vi "myXi_ReshapeArray.vi"(9 "width":i32, 10 "height":i32, 11 "acquisition frame":T1) -> (3 "output array":u16[][](array[numeric]))   [LabVIEW 2018]
uses:
  typedef/AcquisitionFrame.ctl
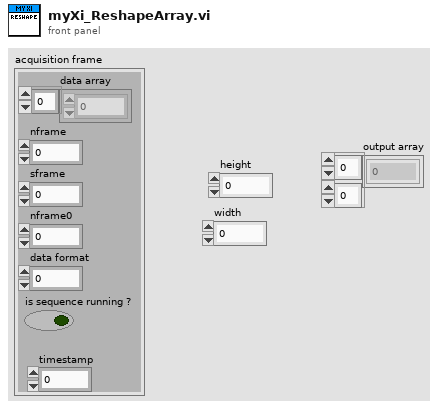
[diagram p1: front panel]
types:
  T1 = typedef "AcquisitionFrame.ctl" = cluster{"data array":u8[], "nframe":i32, "sframe":i32, "nframe0":i32, "data format":i32, "is sequence running ?":bool, "timestamp":dbl}
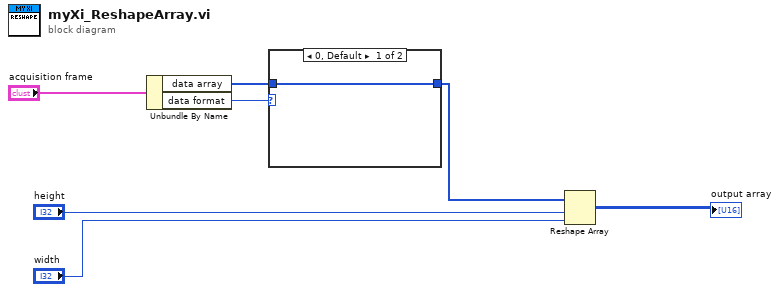
[diagram p0: block diagram]
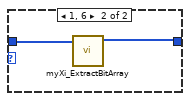
[diagram p2: hidden frame]
diagram:
  n1 = Unbundle By Name("acquisition frame") -> ("data array"=w7:u8[], "data format"=w6:i32)
  n2 = case shown="0, Default" w6 {
    tunnel: w7 -> [w8 w10]
    tunnel: [w8 w9] -> w2
    frame 0, Default {
    }
    frame 1, 6 {
      n3 = call "myXi_ExtractBitArray.vi"("Array"=w10) -> ("(hi.lo) 2"=w9:u16[])  [unwired: 10 in]
    }
  }
  n4 = Reshape Array "Reshape Array"(w2, "height", "width") -> (→"output array":u16[][])
